vi "download_calibration_rm_depth_ahat.vi"(9 "port":u16, 10 "host":string, 11 "path in":path=path "hl2ss_ulm.dll") -> (1 "error":bool, 2 "calibration":T1, 3 "path out":path)   [LabVIEW 2023]
panel:
  in  "calibration":T1
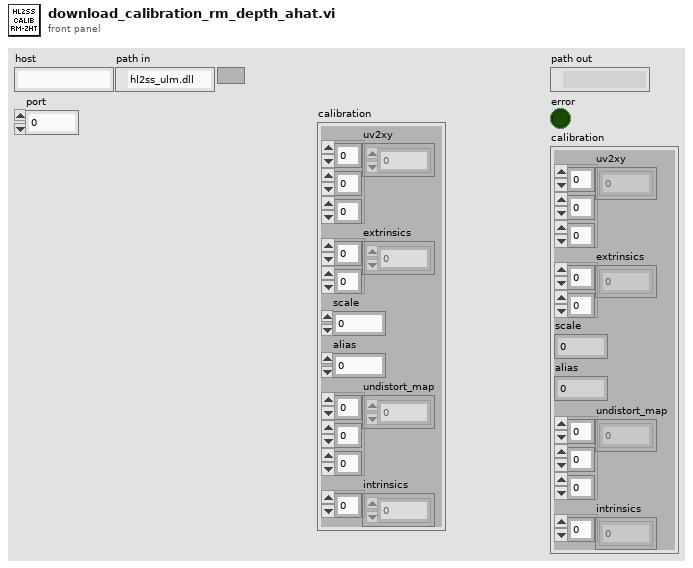
[diagram p1: front panel]
types:
  T1 = cluster{"uv2xy":sgl[][][], "extrinsics":sgl[][], "scale":sgl, "alias":sgl, "undistort_map":sgl[][][], "intrinsics":sgl[]}
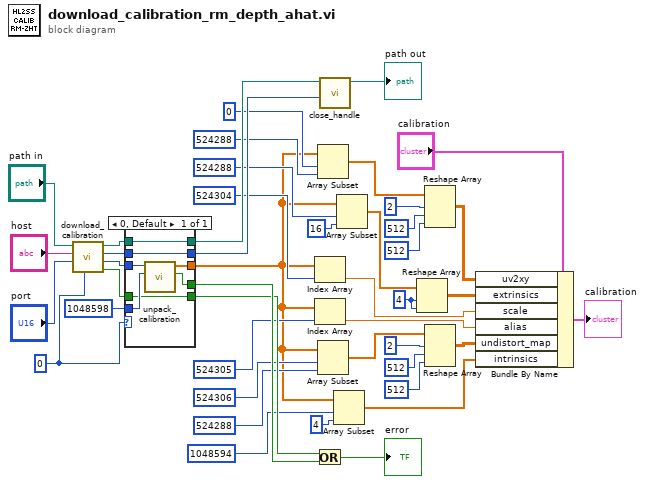
[diagram p0: block diagram]
diagram:
  w5 = 4 ("dimension size")
  w41 = u64 0 ("configuration")
  n1 = call "download_calibration.vi"("configuration"=w41, "port"="port", "host"="host", "path in"="path in") -> ("error"=w30:bool, "calibration"=w39:u64, "calibration_handle"=w37:u64, "path out"=w38:path)  [unwired: 4 in]
  n2 = case shown="0, Default" w41 {
    tunnel: 1048598 ("element_count") -> [w51]
    tunnel: w39 -> [w50]
    tunnel: w38 -> [w49]
    tunnel: w37 -> [w48]
    tunnel: [w49] -> w36
    tunnel: [w48] -> w35
    tunnel: [w47] -> w19
    tunnel: [w46] -> w34
    tunnel: [w45] -> w31
    tunnel: w30 -> [w45]
    frame 0, Default {
      n3 = call "unpack_calibration.vi"("element_count"=w51, "calibration"=w50) -> ("error"=w46:bool, "calibration"=w47:sgl[])  [unwired: 8 in]
    }
  }
  n4 = Index Array(array=w19, index=524304) -> (element=w16:sgl)
  n5 = Index Array(array=w19, index=524305) -> (element=w15:sgl)
  n6 = Or(x=w31, y=w34) -> (x .or. y?=→"error":bool)
  n7 = Array Subset(array=w19, index=0, length=524288) -> (w7:sgl[])
  n8 = Array Subset(array=w19, index=524306, length=524288) -> (w14:sgl[])
  n9 = call "close_handle.vi"("handle"=w35, "path in"=w36) -> ("path out"=→"path out":path)  [unwired: 9 in]
  n10 = Array Subset(array=w19, index=1048594, length=4) -> (w1:sgl[])
  n11 = Array Subset(array=w19, index=524288, length=16) -> (w4:sgl[])
  n12 = Reshape Array(w4, w5, w5) -> (w3:sgl[][])
  n13 = Reshape Array(w7, 2 ("dimension size"), 512 ("dimension size"), 512 ("dimension size")) -> (w6:sgl[][][])
  n14 = Reshape Array(w14, 2 ("dimension size"), 512 ("dimension size"), 512 ("dimension size")) -> (w2:sgl[][][])
  n15 = Bundle By Name(cluster="calibration", "uv2xy"=w6, "extrinsics"=w3, "scale"=w16, "alias"=w15, "undistort_map"=w2, "intrinsics"=w1) -> (→"calibration":T1)
